vi "oscilloscope.vi"() -> ()   [LabVIEW 2021]
uses:
  <vilib>/measure/mascope.llb/Cycle Average and RMS 1 chan.vi
  <vilib>/measure/mascope.llb/Amplitude and Levels 1 chan.vi
  <vilib>/measure/matone.llb/Extract Single Tone Information 1 Chan.vi
  <vilib>/measure/NI_MAPro.lvlib
  <vilib>/measure/NI_MABase.lvlib
panel:
  in  "?":bool
  out "Magnitude difference":dbl
  out "Time diffrence":dbl
  out "cycle RMS":dbl format="%.2g"
  out "cycle average":dbl format="%.2p"
  out "Peak to Peak":dbl format="%.2p"
  in  "Ring":u16(ring) items=["Sine", "Square", "Triangle", "Sawtooth"]
  out "Frequency":dbl
  out "Phase":dbl
  in  "Frequecny":dbl
  in  "Phase":dbl
  out "Amplitude":dbl
  in  "Amplitude":dbl
  out "Oscilloscope":waveform(dbl)(graph)
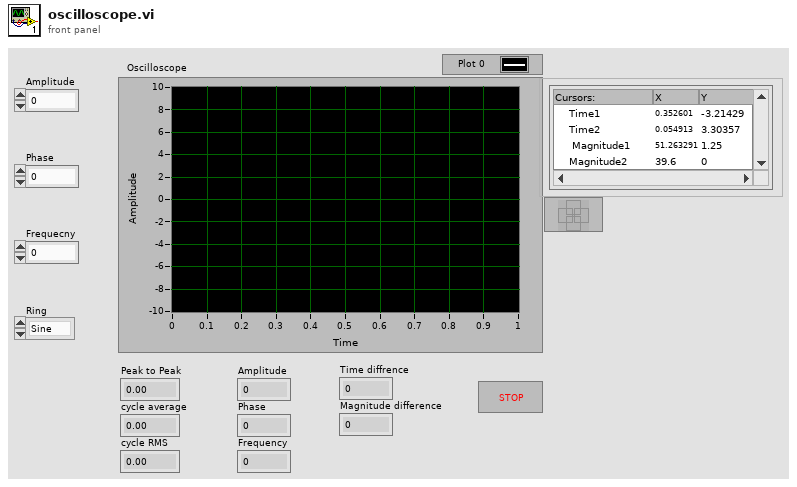
[diagram p1: front panel]
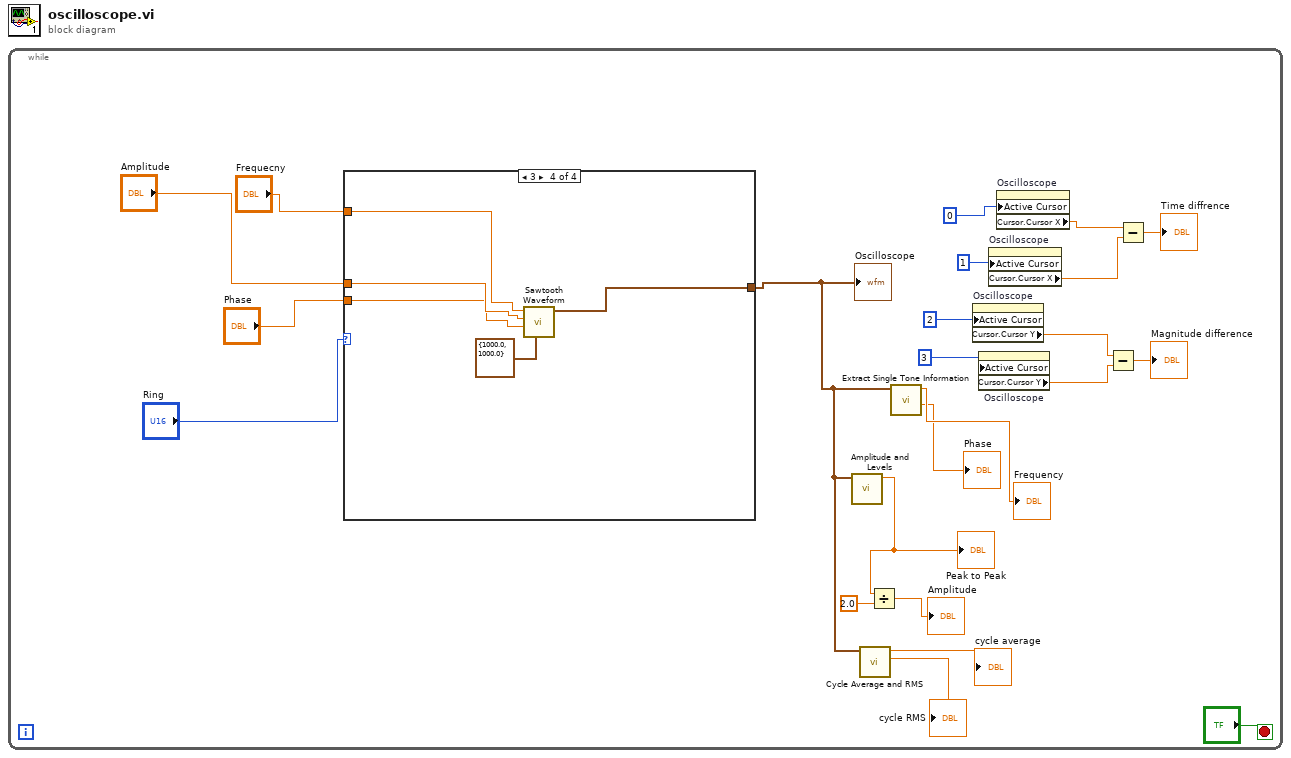
[diagram p0: block diagram]
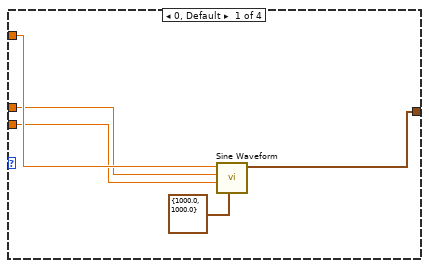
[diagram p2: hidden frame]
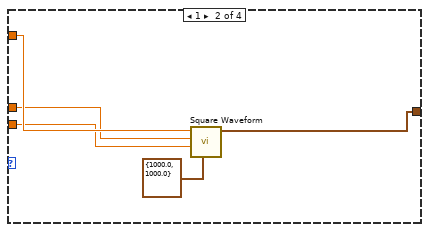
[diagram p3: hidden frame]
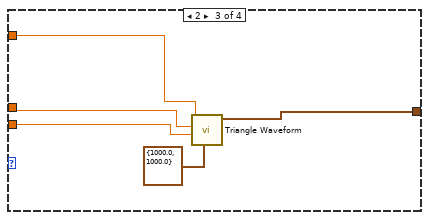
[diagram p4: hidden frame]
diagram:
  n1 = while {
    stop <- "?" stop-if-true
    n2 = case shown="3" "Ring" {
      tunnel: "Frequecny" -> [w28 w33 w38 w43]
      tunnel: "Amplitude" -> [w27 w32 w37 w42]
      tunnel: [w25 w30 w35 w40] -> w14
      tunnel: "Phase" -> [w26 w31 w36 w41]
      frame 0, Default {
        n3 = call <vilib>:"Sine Waveform.vi"("sampling info"=cluster{"Fs":dbl, "#s":dbl} {"Fs"=1000.0, "#s"=1000.0}, "phase"=w26, "amplitude"=w27, "frequency"=w28) -> ("signal out"=w25:waveform(dbl))  [unwired: 6 in, 1 out]
      }
      frame 1 {
        n4 = call <vilib>:"Square Waveform.vi"("sampling info"=cluster{"Fs":dbl, "#s":dbl} {"Fs"=1000.0, "#s"=1000.0}, "phase"=w31, "amplitude"=w32, "frequency"=w33) -> ("signal out"=w30:waveform(dbl))  [unwired: 6 in, 1 out]
      }
      frame 2 {
        n5 = call <vilib>:"Triangle Waveform.vi"("sampling info"=cluster{"Fs":dbl, "#s":dbl} {"Fs"=1000.0, "#s"=1000.0}, "phase"=w36, "amplitude"=w37, "frequency"=w38) -> ("signal out"=w35:waveform(dbl))  [unwired: 6 in, 1 out]
      }
      frame 3 {
        n6 = call <vilib>:"Sawtooth Waveform.vi"("sampling info"=cluster{"Fs":dbl, "#s":dbl} {"Fs"=1000.0, "#s"=1000.0}, "phase"=w41, "amplitude"=w42, "frequency"=w43) -> ("signal out"=w40:waveform(dbl))  [unwired: 6 in, 1 out]
      }
    }
    "Oscilloscope" <- w14
    n7 = call-poly <vilib>:"Amplitude and Levels.vi"("signal in"=w14) -> ("amplitude"=w17:dbl)  [unwired: 7 in, 3 out]
    "Peak to Peak" <- w17
    n8 = call-poly <vilib>:"Cycle Average and RMS.vi"("signal in"=w14) -> ("cycle RMS"=→"cycle RMS":dbl, "cycle average"=→"cycle average":dbl)  [unwired: 7 in, 2 out]
    n9 = Divide(x=w17, y=2.0) -> (x/y=→"Amplitude":dbl)
    n10 = call-poly <vilib>:"Extract Single Tone Information.vi"("time signal in"=w14) -> ("detected phase (deg)"=→"Phase":dbl, "detected frequency"=→"Frequency":dbl)  [unwired: 5 in, 4 out]
    n11 = property on="Oscilloscope" class="WFGraph (strict)"("Active Cursor"=u32 2) -> ("Cursor.Cursor Y"=w4:dbl)  [unwired: 2 in, 2 out]
    n12 = property on="Oscilloscope" class="WFGraph (strict)"("Active Cursor"=u32 3) -> ("Cursor.Cursor Y"=w3:dbl)  [unwired: 2 in, 2 out]
    n13 = property on="Oscilloscope" class="WFGraph (strict)"("Active Cursor"=u32 1) -> ("Cursor.Cursor X"=w8:dbl)  [unwired: 2 in, 2 out]
    n14 = property on="Oscilloscope" class="WFGraph (strict)"("Active Cursor"=u32 0) -> ("Cursor.Cursor X"=w9:dbl)  [unwired: 2 in, 2 out]
    n15 = Subtract(x=w4, y=w3) -> (x-y=→"Magnitude difference":dbl)
    n16 = Subtract(x=w9, y=w8) -> (x-y=→"Time diffrence":dbl)
  }
